vi "CheminDeBase.vi"() -> ()   [LabVIEW 2020]
panel:
  in  "chemin de base":path
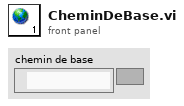
[diagram p1: front panel]
diagram:
